vi "UHR-Fleezers Control (host) - 10.6.vi"() -> ()   [LabVIEW 2011] (continued)
      w2669 = T17 0 items=["Grayscale (U8)", "Grayscale (I16)", "Grayscale (SGL)", "Complex (CSG)", "RGB (U32)", "HSL (U32)", "RGB (U64)"] ("Image Type")
      n1729 = for "Create Greyscale map" {
        N: 256 -> [_]
        tunnel: [w2675] -> w2658 mode=indexing
        workers-P: _ -> [_]
        i -> [w2678]
        n1730 = To Unsigned Byte Integer(number=w2678) -> (unsigned 8bit integer=w2674:u8)
        n1731 = Join Numbers(hi=w2674, lo=w2674) -> ((hi.lo)=w2677:u16)
        n1732 = Join Numbers(hi=w2674, lo=w2674) -> ((hi.lo)=w2676:u16)
        n1733 = Join Numbers(hi=w2677, lo=w2676) -> ((hi.lo)=w2675:u32)
      }
      n1734 = call "IMAQ Create"("Image Name"="Scaled video", "Image Type"=w2661) -> ("New Image"=w2660:T2)  [unwired: 2 in, 2 out]
      n1735 = call "IMAQ Create"("Image Name"="Main video", "Image Type"=w2669) -> ("New Image"=w2670:T2)  [unwired: 2 in, 2 out]
      n1736 = node-c288(0 ("Processor")) -> (w2668:T21)  [unwired: 3 out]
      n1737 = Initialize Array(u32 0 ("Window Number (0...15)"), 480 ("dimension size"), 640 ("dimension size")) -> (w2663:u32[][])
      n1738 = timed-loop {
        tunnel: w2673 -> [w2695]
        tunnel: [w2694] -> w2672
        tunnel: w2670 -> [w2693]
        timing: w2668 -> [_]
        timing-out: [_] -> w2667
        tunnel: w2663 -> [w2682]
        tunnel: w2660 -> [w2680]
        tunnel: w2658 -> [w2679]
        stop <- w2681 stop-if-true
        # "This block performs the \nactual image capture."
        n1739 = node-c288() -> ()  [unwired: 2 out]
        n1740 = local read "Stop All"() -> (w2681:bool)
        n1741 = Reciprocal(x="Video Capture Rate (Hz)") -> (1/x=w2685:dbl)
        n1742 = Multiply(x=w2685, y=1000.0) -> (x*y=w2683:dbl)
        n1743 = call "DMR_ImageRequestWaitFor.vi"("queue number IN"=0, "timeout(ms) IN"=500, "driver handle IN"=w2695) -> ("error code OUT"=w2699:i32, "request number OUT"=w2696:i32, "driver handle OUT"=w2697:i32)
        n1744 = feedback #1(T32 refnum ("Avi Refnum")) -> (w2687:T32)
        n1745 = case shown="True" "New Video File" {
          tunnel: [T32 refnum ("Avi Refnum") w2716] -> w2689
          tunnel: [FALSE TRUE] -> w2690
          tunnel: w2687 -> [_ w2712]
          frame False {
          }
          frame True {
            n1746 = call "Create new save file.vi"("Ext"=".avi" ("string"), "Index In"="Video Index") -> ("Path Out"=w2708:path, "Index Out"=w2709:dbl)  [unwired: 1 in]
            "Path Out" <- w2708
            n1747 = Not Equal?(x=w2712, y=T32 refnum ("Avi Refnum")) -> (x != y?=w2713:bool)
            n1748 = Increment(x=w2709) -> (x+1=w2718:dbl)
            n1749 = case shown="True" w2713 {
              tunnel: w2712 -> [_ w2719]
              frame False {
              }
              frame True {
                n1750 = call "IMAQ AVI Close"("Avi Refnum"=w2719) -> ()  [unwired: 1 in, 10 out]
              }
            }
            n1751 = local write "Video Index"(w2718) -> ()
            n1752 = call "IMAQ AVI Create"("Frames Per Second"=u32 30, "AVI Path"=w2708) -> ("Avi Refnum"=w2716:T32)  [unwired: 5 in, 4 out]
          }
        }
        n1753 = Equal To 0?(x=w2699) -> (x = 0?=w2698:bool)
        n1754 = Select(t=w2689, s=w2690, f=w2687) -> (s? t:f=w2688:T32)
        n1755 = feedback-in #1(w2688) -> ()
        n1756 = case shown="True" w2698 {
          tunnel: w2697 -> [w2720 w2745]
          tunnel: w2696 -> [_ w2744]
          tunnel: [w2720 w2741] -> w2694
          tunnel: w2693 -> [_ w2725]
          tunnel: w2682 -> [_ w2729]
          tunnel: w2688 -> [_ w2727]
          tunnel: w2680 -> [_ w2722]
          tunnel: w2679 -> [_ w2721]
          frame False {
          }
          frame True {
            w2735 = u32 0 ("X-offset IN")
            n1757 = call "DMR_GetImageRequestBufferData.vi"("driver handle IN"=w2745, "request number IN"=w2744) -> ("width OUT"=w2734:i32, "height OUT"=w2733:i32, "driver handle OUT"=w2740:i32, "request number OUT"=w2739:i32, "bytes per pixel OUT"=w2736:i32)  [unwired: 13 out]
            n1758 = call "DMR_GetImageRequestBufferImageData.vi"("driver handle IN"=w2740, "request number IN"=w2739, "bytes per pixel IN"=w2736, "X-offset IN"=w2735, "Y-offset IN"=w2735, "height IN"=w2733, "width IN"=w2734) -> ("driver handle OUT"=w2738:u32, "request number OUT"=w2737:u32, "image OUT"=w2730:u32[][])  [unwired: 10 out]
            n1759 = call "DMR_ImageRequestUnlock.vi"("request number IN"=w2737, "driver handle IN"=w2738) -> ("driver handle OUT"=w2743:i32)  [unwired: 1 in, 2 out]
            n1760 = case shown="True" "Averaging" {
              tunnel: w2730 -> [w2781 w2786]
              tunnel: [w2781 w2785] -> w2726
              tunnel: w2729 -> [_ w2783]
              frame False {
              }
              frame True {
                (unwired) 1
                w2791 = 1
                n1761 = feedback #2(w2783) -> (w2782:u32[][])
                n1762 = Add(x=w2786, y=w2782) -> (x+y=w2787:u32[][])
                n1763 = Select(t=w2783, s="Reset Averaging", f=w2787) -> (s? t:f=w2789:u32[][])
                n1764 = feedback-in #2(w2789) -> ()
                n1765 = feedback #3(w2791) -> (w2784:i32)
                n1766 = Divide(x=w2787, y=w2784) -> (x/y=w2788:dbl[][])
                n1767 = Increment(x=w2784) -> (x+1=w2792:i32)
                n1768 = To Unsigned Long Integer(number=w2788) -> (unsigned 32bit integer=w2785:u32[][])
                n1769 = Select(t=w2791, s="Reset Averaging", f=w2792) -> (s? t:f=w2790:i32)
                n1770 = feedback-in #3(w2790) -> ()
              }
            }
            n1771 = call "DMR_ImageRequestSingle.vi"("request control IN"=0, "driver handle IN"=w2743) -> ("driver handle OUT"=w2741:i32)  [unwired: 3 out]
            n1772 = disable-structure shown="Disabled" {
              disable-tunnel: w2726 -> [w2758 _]
              disable-tunnel: w2722 -> [w2757 _]
              frame Disabled {
                n1773 = To Double Precision Float(number=w2758) -> (double precision float=w2756:dbl[][])
                n1774 = In Range and Coerce(upper limit="Intensity Upper", x=w2756, lower limit="Intensity Lower") -> (coerced(x)=w2755:dbl[][])  [unwired: 1 out]
                n1775 = Subtract(x="Intensity Upper", y="Intensity Lower") -> (x-y=w2752:dbl)
                n1776 = Subtract(x=w2755, y="Intensity Lower") -> (x-y=w2753:dbl[][])
                n1777 = Divide(x=w2753, y=w2752) -> (x/y=w2754:dbl[][])
                n1778 = Multiply(x=255.0, y=w2754) -> (x*y=w2750:dbl[][])
                n1779 = To Unsigned Byte Integer(number=w2750) -> (unsigned 8bit integer=w2759:u8[][])
                n1780 = call "IMAQ ArrayToImage"("Image Pixels (U8)"=w2759, "Image"=w2757) -> ("Image Out"=w2746:T2)  [unwired: 4 in, 5 out]
                n1781 = First Call?() -> (First Call?: T/F=w2747:bool)
                n1782 = case shown="True" w2747 {
                  tunnel: w2746 -> [w2760 w2771]
                  frame False {
                    n1783 = flat-sequence {
                      tunnel: w2760 -> [w2766]
                      frame #0 {
                        w2763 = FALSE ("Get/Set Status? (Set)")
                        w2762 = 0 ("Window Number (0...15)")
                        n1784 = call "IMAQ WindSize"("Get/Set Status? (Set)"=w2763, "Window Number"=w2762) -> ("Width & Height out"=→"Window Size":cluster{"Width":i32, "Height":i32})  [unwired: 4 in, 2 out]
                        n1785 = call "IMAQ WindMove"("Window Number (0...15)"=w2762, "Get/Set Status? (Set)"=w2763) -> ("Coordinates (screen)"=→"Window Position":cluster{"X Position":i32, "Y Position":i32})  [unwired: 3 in, 1 out]
                        n1786 = call "IMAQ WindDraw"("Resize to Image Size? (Y)"=FALSE, "Window Number (0...15)"=w2762, "Image"=w2766) -> ()  [unwired: 7 in, 2 out]
                      }
                      frame #1 {
                        n1787 = call "IMAQ WindZoom 2"("Center Point"="Center Point", "Zoom to Fit? (False)"=FALSE, "Zoom Factor"="Zoom Factor") -> ()  [unwired: 5 in, 4 out]
                      }
                    }
                  }
                  frame True {
                    n1788 = flat-sequence {
                      tunnel: w2771 -> [w2774]
                      tunnel: [w2772] -> w2770
                      tunnel: w2770 -> [w2776]
                      frame #0 {
                        w2773 = TRUE ("Resize to Image Size? (Y)")
                        w2772 = 0 ("Window Number (0...15)")
                        n1789 = call "IMAQ WindNonTearing"("Window Number"=w2772, "NonTearing? (True)"=w2773) -> ()  [unwired: 8 in, 2 out]
                        n1790 = call "IMAQ WindDraw"("Resize to Image Size? (Y)"=w2773, "Window Number (0...15)"=w2772, "Image"=w2774) -> ()  [unwired: 7 in, 2 out]
                      }
                      frame #1 {
                        n1791 = call "IMAQ WindSize"("Scrollbars? (N)"=FALSE, "Width & Height"="Initial Window Size", "Window Number"=w2776) -> ()  [unwired: 3 in, 3 out]
                        n1792 = call "IMAQ WindMove"("Window Number (0...15)"=w2776, "Coordinates (screen)"="Initial Window Position") -> ()  [unwired: 3 in, 2 out]
                      }
                    }
                  }
                }
              }
              frame Enabled {
              }
            }
            n1793 = To Unsigned Byte Integer(number=w2726) -> (unsigned 8bit integer=w2724:u8[][])
            n1794 = call "IMAQ ArrayToImage"("Image Pixels (U8)"=w2724, "Image"=w2725) -> ("Image Out"=w2723:T2)  [unwired: 4 in, 5 out]
            "Primary Video Display" <- w2723
            n1795 = case shown="True" "Save Video" {
              tunnel: w2727 -> [_ w2780]
              tunnel: w2723 -> [_ w2779]
              frame False {
              }
              frame True {
                n1796 = call "IMAQ AVI Write Frame"("Image"=w2779, "Avi Refnum"=w2780) -> ()  [unwired: 2 in, 8 out]
              }
            }
            n1797 = case shown="True" "Save Image" {
              tunnel: w2724 -> [_ w2795]
              tunnel: w2721 -> [_ w2794]
              frame False {
              }
              frame True {
                n1798 = call <vilib>:"Flatten Pixmap.vi"("colors"=w2794, "8-bit pixmap"=w2795) -> ("image data"=w2801:T33)  [unwired: 4 in, 5 out]
                n1799 = call "Create new save file.vi"("Insert"="video_frame_" ("string"), "Ext"=".bmp" ("string"), "Index In"="Image Index") -> ("Path Out"=w2797:path, "Index Out"=w2802:dbl)
                n1800 = Increment(x=w2802) -> (x+1=w2796:dbl)
                n1801 = local write "Image Index"(w2796) -> ()
                n1802 = call <vilib>:"Write BMP File.vi"("image data"=w2801, "path to BMP file"=w2797) -> ()  [unwired: 1 in, 9 out]
              }
            }
          }
        }
        n1803 = node-c288(w2683) -> ()  [unwired: 1 out]
      }
      n1804 = node-c288(w2667) -> ()  [unwired: 1 out]
      n1805 = call "DMR_CloseDevice.vi"("driver handle IN"=w2672) -> ()  [unwired: 1 in, 4 out]
    }
    frame #4 {
      n1806 = call "DMR_Close.vi"() -> ()  [unwired: 1 out]
    }
  }
  n1807 = node-c288(i64 1 ("Period"), 1 ("Processor")) -> (w175:T21)  [unwired: 2 out]
  n1808 = timed-loop "Acquire Data" {
    tunnel: w50 -> [w3101]
    tunnel: w49 -> [w3100]
    tunnel: [w3130] -> w270
    tunnel: [w3125] -> w268
    timing: w175 -> [_]
    timing-out: [_] -> w174
    tunnel: w69 -> [w2938]
    stop <- "Stop All" stop-if-true
    w2853 = "Initialize"
    w2923 = "NI_ChannelName" ("name")
    n1809 = node-c288() -> ()  [unwired: 2 out]
    n1810 = First Call?() -> (First Call?: T/F=w2888:bool)
    n1811 = Or(x="Reset", y=w2888) -> (x .or. y?=w2889:bool)
    n1812 = local read "Flushing P1"() -> (w2807:bool)
    n1813 = case "Reset data stream" shown="True" w2889 {
      tunnel: w3101 -> [w4106 w4114]
      tunnel: w3100 -> [w4105 w4113]
      tunnel: [w4106 w4108] -> w3096
      tunnel: [w4105 w4107] -> w3095
      frame False {
      }
      frame True {
        w4111 = TRUE ("AI to FIFO")
        n1814 = local write "Overflow (data lost)"(FALSE ("Overflow (data lost)")) -> ()
        n1815 = call "reset FPGA DMA.vi"("error in"=w4113, "FPGA VI Reference In"=w4114) -> ("error out"=w4109:errorcluster, "FPGA VI Reference Out"=w4110:T19)
        n1816 = xnode "Read/Write Control"("FPGA VI Reference In"=w4110, "error in"=w4109, "AI to FIFO"=w4111, "APD to FIFO"=w4111) -> ("FPGA VI Reference Out"=w4108:T19, "error out"=w4107:errorcluster)
      }
    }
    n1817 = case shown="True" w2807 {
      frame False {
      }
      frame True {
        n1818 = local read "Flush rate (uL/m) P1"() -> (w3147:dbl)
        n1819 = local read "HP1 Flush Time (s)"() -> (w3156:dbl)
        n1820 = local read "DMA Update Period (s)"() -> (w3150:dbl)
        n1821 = Divide(x=w3147, y=60.0) -> (x/y=w3148:dbl)
        n1822 = Divide(x=w3156, y=w3150) -> (x/y=w3145:dbl)
        n1823 = feedback #4(0) -> (w3154:i32)
        n1824 = Increment(x=w3154) -> (x+1=w3144:i32)
        n1825 = Greater?(x=w3144, y=w3145) -> (0:w3153:bool)
        n1826 = Compound Arithmetic op=MULTIPLY(w3150, w3144, w3148) -> (→"P1 Flush Volume (uL)":dbl)
        n1827 = Divide(x=w3144, y=w3145) -> (x/y=→"P1 Flushing Bar":dbl)
        n1828 = case shown="True" w3153 {
          tunnel: w3144 -> [w3157 _]
          tunnel: [w3157 0] -> w3152
          frame False {
          }
          frame True {
            w3158 = FALSE ("Flushing P1")
            n1829 = local write "Inject Pump 1"(w3158) -> ()
            n1830 = local write "Flushing P1"(w3158) -> ()
            n1831 = property on="Clear Volume P1" class="Bool (strict)"("Val(Sgnl)"=TRUE ("Value (Signaling)")) -> ()  [unwired: 2 in, 2 out]
          }
        }
        n1832 = feedback-in #4(w3152) -> ()
      }
    }
    n1833 = Or(x="Start AOD Scan", y="Trap Raster Scan") -> (x .or. y?=w3046:bool)
    n1834 = case "Start AOM raster scan" shown="True" w3046 {
      tunnel: w3096 -> [w3956 w3966]
      tunnel: w3095 -> [w3955 w3965]
      tunnel: [w3956 w3959] -> w3094
      tunnel: [w3955 w3958] -> w3093
      frame False {
      }
      frame True {
        n1835 = case shown="True" "Restart DMA? (AOD)" {
          tunnel: [w4004 w4006] -> w3960
          tunnel: [w4003 w4005] -> w3961
          tunnel: w3966 -> [w4004 w4008]
          tunnel: w3965 -> [w4003 w4007]
          frame False {
          }
          frame True {
            n1836 = local write "Overflow (data lost)"(FALSE ("Overflow (data lost)")) -> ()
            n1837 = call "reset FPGA DMA.vi"("error in"=w4007, "FPGA VI Reference In"=w4008) -> ("error out"=w4005:errorcluster, "FPGA VI Reference Out"=w4006:T19)
          }
        }
        n1838 = local write "Trap Raster Scan"(FALSE ("Trap Raster Scan")) -> ()
        n1839 = case shown="True" "Move MCL Also?" {
          tunnel: w3961 -> [w3969 w3998]
          tunnel: w3960 -> [w3970 w3999]
          tunnel: [w3968 w4002] -> w3959
          tunnel: [w3967 w4001] -> w3958
          frame False {
            w3971 = TRUE ("AI to FIFO")
            n1840 = xnode "Read/Write Control"("FPGA VI Reference In"=w3970, "error in"=w3969, "AI to FIFO"=w3971, "APD to FIFO"=w3971, "Start scan"=w3971) -> ("FPGA VI Reference Out"=w3968:T19, "error out"=w3967:errorcluster)
          }
          frame True {
            w3995 = FALSE ("1D or 2D Scan?")
            w4000 = TRUE ("AI to FIFO")
            # "Count for MCL loop"
            # "N total cycles"
            # "N steps"
            # "V_int"
            n1841 = local read "Scan Range (nm)"() -> (w3977:dbl)
            n1842 = local read "Number of F/B Scans (AOD)"() -> (w3994:u16)
            n1843 = Sign(1:w3977) -> (0:w3976:dbl)
            n1844 = Compound Arithmetic op=MULTIPLY(w3977, "MCL Step Position Ratio", "MCL/AOM Scale Tweak") -> (w3981:dbl)
            n1845 = Negate(x=w3976) -> (-x=w3973:dbl)
            n1846 = Multiply(x=w3973, y="MCL Step Increment (V_int)") -> (x*y=w3975:dbl)
            n1847 = Divide(x=w3981, y="MCL X Cal (nm/V)") -> (x/y=w3987:dbl)
            n1848 = Multiply(x=32767.0 ("y"), y=w3987) -> (x*y=w3993:dbl)
            n1849 = local read "Total Counts (ticks)"() -> (w3978:u32)
            n1850 = local read "Cycles/step (AOD)"() -> (w3989:u64)
            n1851 = local read "Scan steps (AOD)"() -> (w3990:u64)
            n1852 = Divide(x=w3993, y=10.0) -> (x/y=w3986:dbl)
            n1853 = Divide(x=w3986, y="MCL Step Increment (V_int)") -> (x/y=w3984:dbl)
            n1854 = Absolute Value(x=w3984) -> (abs(x)=w3972:dbl)
            n1855 = Compound Arithmetic op=MULTIPLY(w3990, w3989, w3978) -> (w3985:u64)
            n1856 = local write "wait to reset values"(w4000) -> ()
            n1857 = local write "MCL Scanning"(w4000) -> ()
            n1858 = Divide(x=w3985, y=w3972) -> (x/y=w3982:dbl)
            "MCL Count" <- w3982
            n1859 = xnode "Read/Write Control"("FPGA VI Reference In"=w3999, "error in"=w3998, "Scan steps (MCL)"=w3972, "Number of scans (MCL)"=w3994, "Cycles per step (MCL)"=u64 1, "Scan freq.  increment (MCL)"=w3975, "1D or 2D Scan?"=w3995, "MCL Scan Axis"=w3995, "Cont. Scan (MCL)"=w3995, "MCL count"=w3982) -> ("FPGA VI Reference Out"=w3997:T19, "error out"=w3996:errorcluster)
            n1860 = xnode "Read/Write Control"("FPGA VI Reference In"=w3997, "error in"=w3996, "AI to FIFO"=w4000, "APD to FIFO"=w4000, "Start scan"=w4000, "Start scan (MCL)"=w4000) -> ("FPGA VI Reference Out"=w4002:T19, "error out"=w4001:errorcluster)
          }
        }
        "Raster Scanning..." <- TRUE ("Scanning...")
      }
    }
    n1861 = local read "Flushing P3"() -> (w2808:bool)
    n1862 = case "Keep track of when Harvard Pump 3 is done flushing" shown="True" w2808 {
      frame False {
      }
      frame True {
        n1863 = local read "Flush rate (uL/m) P3"() -> (w3164:dbl)
        n1864 = local read "DMA Update Period (s)"() -> (w3166:dbl)
        n1865 = local read "HP3 Flush Time (s)"() -> (w3173:dbl)
        n1866 = Divide(x=w3164, y=60.0) -> (x/y=w3162:dbl)
        n1867 = feedback #5(0) -> (w3171:i32)
        n1868 = Increment(x=w3171) -> (x+1=w3165:i32)
        n1869 = Divide(x=w3173, y=w3166) -> (x/y=w3167:dbl)
        n1870 = Greater?(x=w3165, y=w3167) -> (0:w3170:bool)
        n1871 = Compound Arithmetic op=MULTIPLY(w3166, w3165, w3162) -> (→"P3 Flush Volume (uL)":dbl)
        n1872 = case shown="True" w3170 {
          tunnel: w3165 -> [w3174 _]
          tunnel: [w3174 0] -> w3169
          frame False {
          }
          frame True {
            w3175 = FALSE ("Flushing P3")
            n1873 = local write "Inject Pump 3"(w3175) -> ()
            n1874 = local write "Flushing P3"(w3175) -> ()
            n1875 = property on="Clear Volume P3" class="Bool (strict)"("Val(Sgnl)"=TRUE ("Value (Signaling)")) -> ()  [unwired: 2 in, 2 out]
          }
        }
        n1876 = feedback-in #5(w3169) -> ()
        n1877 = Divide(x=w3165, y=w3167) -> (x/y=→"P3 Flushing Bar":dbl)
      }
    }
    n1878 = And(x="Save scans", y=w3046) -> (x .and. y?=w3092:bool)
    n1879 = Compound Arithmetic op=OR("Start MCL Scan", "Confocal Image", "Confocal Linescan") -> (w3044:bool)
    n1880 = And(x="Save Data (MCL)", y=w3044) -> (x .and. y?=w3091:bool)
    n1881 = case "Start MCL raster scan" shown="True" w3044 {
      tunnel: w3094 -> [w3573 w3589]
      tunnel: w3093 -> [w3572 w3588]
      tunnel: [w3573 w3584] -> w2936
      tunnel: [w3572 w3583] -> w2935
      tunnel: [FALSE w3582] -> w3077
      tunnel: "Start MCL Scan" -> [_ w3577]
      tunnel: "Confocal Image" -> [_ w3576]
      tunnel: "Confocal Linescan" -> [_ _]
      frame False {
      }
      frame True {
        w3582 = TRUE
        n1882 = case shown="True" "Restart DMA? (MCL)" {
          tunnel: [w3634 w3636] -> w3587
          tunnel: [w3633 w3635] -> w3586
          tunnel: w3589 -> [w3634 w3639]
          tunnel: w3588 -> [w3633 w3638]
          frame False {
          }
          frame True {
            n1883 = call "reset FPGA DMA.vi"("error in"=w3638, "FPGA VI Reference In"=w3639) -> ("error out"=w3635:errorcluster, "FPGA VI Reference Out"=w3636:T19)
            n1884 = local write "Overflow (data lost)"(FALSE ("Overflow (data lost)")) -> ()
          }
        }
        n1885 = case shown="False" w3577 {
          selector: w3577 -> [_ w3593]
          tunnel: w3576 -> [w3592 _]
          tunnel: [w3592 w3593] -> w3575
          frame False {
            n1886 = property on="2D or 1D Scan" class="Bool (strict)"("Val(Sgnl)"=w3592) -> ()  [unwired: 2 in, 2 out]
            n1887 = property on="Confocal Image" class="Bool (strict)"("Value"=FALSE ("Start Confocal Map")) -> ()  [unwired: 2 in, 2 out]
          }
          frame True {
          }
        }
        n1888 = local write "MCL Scanning"(w3582) -> ()
        n1889 = local read "AO1"() -> (w3579:dbl)
        n1890 = local read "AO2"() -> (w3578:dbl)
        n1891 = case shown="True" "Center Scan" {
          tunnel: w3587 -> [w3600 w3632]
          tunnel: w3586 -> [w3599 w3631]
          tunnel: [w3598 w3630] -> w3584
          tunnel: [w3597 w3629] -> w3583
          tunnel: [w3595 w3616] -> w3581
          tunnel: [w3594 w3615] -> w3580
          tunnel: w3579 -> [w3595 w3621]
          tunnel: w3578 -> [w3594 w3624]
          tunnel: w3575 -> [_ _]
          frame False {
            w3596 = TRUE ("AI to FIFO")
            n1892 = xnode "Read/Write Control"("FPGA VI Reference In"=w3600, "error in"=w3599, "AI to FIFO"=w3596, "APD to FIFO"=w3596, "Start scan (MCL)"=w3596) -> ("FPGA VI Reference Out"=w3598:T19, "error out"=w3597:errorcluster)
          }
          frame True {
            w3628 = TRUE ("AI to FIFO")
            n1893 = local read "Scan steps (MCL)"() -> (w3607:u64)
            n1894 = local read "Scan lines (y)"() -> (w3603:u64)
            n1895 = local read "Fast Scan Dir"() -> (w3614:bool)
            n1896 = local read "Actual MCL Inc (V)"() -> (w3604:dbl)
            n1897 = Decrement(x=w3603) -> (x-1=w3602:u64)
            n1898 = Decrement(x=w3607) -> (x-1=w3606:u64)
            n1899 = Multiply(x=w3604, y=w3602) -> (x*y=w3601:dbl)
            n1900 = Divide(x=w3601, y=2.0) -> (x/y=w3611:dbl)
            n1901 = Multiply(x=w3604, y=w3606) -> (x*y=w3605:dbl)
            n1902 = Divide(x=w3605, y=2.0) -> (x/y=w3610:dbl)
            n1903 = Select(t=w3610, s=w3614, f=w3611) -> (s? t:f=w3609:dbl)
            n1904 = Select(t=w3611, s=w3614, f=w3610) -> (s? t:f=w3613:dbl)
            n1905 = Subtract(x=w3621, y=w3613) -> (x-y=w3612:dbl)
            n1906 = Subtract(x=w3624, y=w3609) -> (x-y=w3608:dbl)
            n1907 = local read "2D or 1D Scan"() -> (w3626:bool)
            n1908 = Not(x=w3614) -> (.not. x?=w3620:bool)
            n1909 = Not(x=w3626) -> (.not. x?=w3622:bool)
            n1910 = And(x=w3614, y=w3622) -> (x .and. y?=w3623:bool)
            n1911 = And(x=w3622, y=w3620) -> (x .and. y?=w3625:bool)
            n1912 = Select(t=w3624, s=w3625, f=w3608) -> (s? t:f=w3615:dbl)
            n1913 = Select(t=w3621, s=w3623, f=w3612) -> (s? t:f=w3616:dbl)
            n1914 = call "Volt to I16.vi"("Voltage In"=w3616) -> ("I16 Voltage Out"=w3619:i16)
            n1915 = call "Volt to I16.vi"("Voltage In"=w3615) -> ("I16 Voltage Out"=w3618:i16)
            n1916 = xnode "Read/Write Control"("FPGA VI Reference In"=w3632, "error in"=w3631, "AI to FIFO"=w3628, "APD to FIFO"=w3628, "Start scan (MCL)"=w3628, "AO1"=w3619, "AO2"=w3618) -> ("FPGA VI Reference Out"=w3630:T19, "error out"=w3629:errorcluster)
          }
        }
        "Initial Y" <- w3581
        "Initial X" <- w3580
        n1917 = local write "Tab Control 6"(T3."Imaging" ("Tab Control 6")) -> ()
        "wait to reset values" <- w3582
      }
    }
    n1918 = local read "Trap Pos Elements/DMA read"() -> (w2932:u32)
    n1919 = local read "Trap AI Elements/DMA read"() -> (w3007:u32)
    n1920 = local read "APD Elements/DMA read"() -> (w2973:u32)
    n1921 = xnode "Get APD Data"("FPGA VI Reference In"=w2936, "error in"=w2935, "Number of Elements"=w2973, "Timeout (ms)"=-1) -> ("Data"=w2972:u32[], "Elements Remaining"=→"APD FIFO Elements Remaining":u32)  [unwired: 2 out]
    n1922 = xnode "Invoke Method"("FPGA VI Reference In"=w2936, "error in"=w2935, "Number of Elements"=w2932, "Timeout (ms)"=-1) -> ("Data"=w2895:u16[], "Elements Remaining"=→"Trap Pos FIFO El Remaining":u32)  [unwired: 2 out]
    n1923 = xnode "Get Trap Data"("FPGA VI Reference In"=w2936, "error in"=w2935, "Number of Elements"=w3007, "Timeout (ms)"=-1 ("Timeout")) -> ("FPGA VI Reference Out"=w2829:T19, "error out"=w2828:errorcluster, "Data"=w2896:i16[], "Elements Remaining"=w3138:u32)
    "FIFO El. Rem." <- w3138
    n1924 = local read "Trap AI FIFO Depth"() -> (w3140:u32)
    n1925 = Subtract(x=w3140, y=w3007) -> (x-y=w3139:u32)
    n1926 = Decimate 1D Array(w2895) -> (w2892:u16[], w2894:u16[], w2893:u16[])
    n1927 = Divide(x=w3138, y=w3139) -> (x/y=w3137:dbl)
    "Buffer Status" <- w3137
    n1928 = To Unsigned Long Integer(number=w2892) -> (unsigned 32bit integer=w2891:u32[])
    n1929 = Join Numbers(hi=w2894, lo=w2893) -> ((hi.lo)=w2890:u32[])
    n1930 = Equal?(x=w3137, y=1.0) -> (x = y?=w3135:bool)
    n1931 = Join Numbers(hi=w2891, lo=w2890) -> ((hi.lo)=w2884:u64[])
    n1932 = call "IR AOM word to freq - vec.vi"("Frequency Word In (double vec)"=w2884) -> ("Frequency Out"=w2931:dbl[])
    n1933 = case "Alert buffer overflow" shown="True" w3135 {
      frame False {
      }
      frame True {
        n1934 = call <vilib>:"Beep.vi"() -> ()  [unwired: 3 in, 9 out]
        "Overflow (data lost)" <- TRUE ("Overflow (data lost)")
      }
    }
    n1935 = Decimate 1D Array(w2931) -> (w2930:dbl[], w2929:dbl[])
    n1936 = Build Array(w2930, w2929) -> (w2928:dbl[][])
    n1937 = local read "Trap Sets"() -> (w3006:u32)
    n1938 = case "Deinterlace trap data, average down PSD" shown="2" w3006 {
      tunnel: w2896 -> [w3669 w3734]
      tunnel: [w3666 w3731] -> w2999
      tunnel: [w3669 w3733] -> w2887
      tunnel: "Detector Type" -> [w3668 w3729]
      tunnel: [w3667 w3732] -> w2998
      tunnel: [w3665 w3730] -> w3112
      frame 1, Default {
        n1939 = Divide(x=w3669, y=3276.7) -> (x/y=w3670:dbl[])
        n1940 = Decimate 1D Array(w3670) -> (w3679:dbl[], w3678:dbl[], w3677:dbl[], w3676:dbl[], w3675:dbl[], w3674:dbl[], w3673:dbl[], w3672:dbl[])
        n1941 = case shown="\"IR-QPD + PSD + FB-QPD position\"" w3668 {
          tunnel: w3679 -> [w3703 w3728]
          tunnel: w3678 -> [w3702 w3727]
          tunnel: w3677 -> [w3687 w3705]
          tunnel: w3676 -> [w3688 w3715]
          tunnel: w3675 -> [w3701 w3726]
          tunnel: w3674 -> [w3700 w3725]
          tunnel: w3673 -> [w3684 w3706]
          tunnel: w3672 -> [w3683 w3704]
          tunnel: [w3682 w3712] -> w3667
          tunnel: [w3681 w3711] -> w3666
          tunnel: [w3680 w3710] -> w3665
          frame "IR-QPD + PSD + FB-QPD", Default {
            w3680 = 0  # Channel pattern
            n1942 = Divide(x=w3703, y=w3688) -> (x/y=w3690:dbl[])
            n1943 = Divide(x=w3702, y=w3688) -> (x/y=w3689:dbl[])
            n1944 = Divide(x=w3701, y=w3684) -> (x/y=w3686:dbl[])
            n1945 = Divide(x=w3700, y=w3683) -> (x/y=w3685:dbl[])
            n1946 = Build Array(w3690, w3689, w3688, w3687, w3686, w3685, w3684, w3683) -> (w3681:dbl[][])
            n1947 = Bundle("T1 Y", "T1 X", "T1 Sum", "FB Sum", "PSD Y", "PSD X", "PSD Y Sum", "PSD X Sum") -> (w3699:T40)  [unwired: 1 out]
            n1948 = Cluster To Array(cluster=w3699) -> (array=w3682:string[])
          }
          frame "IR-QPD + PSD + FB-QPD position" {
            w3710 = 3  # Channel pattern
            n1949 = Negate(x=w3706) -> (-x=w3707:dbl[])
            n1950 = Divide(x=w3728, y=w3715) -> (x/y=w3717:dbl[])
            n1951 = Divide(x=w3727, y=w3715) -> (x/y=w3716:dbl[])
            n1952 = Divide(x=w3726, y=w3706) -> (x/y=w3714:dbl[])
            n1953 = Divide(x=w3725, y=w3707) -> (x/y=w3713:dbl[])
            n1954 = Build Array(w3717, w3716, w3715, w3704, w3705, w3714, w3713, w3706) -> (w3711:dbl[][])
            n1955 = Bundle("T1 Y", "T1 X", "T1 Sum", "FB X", "FB Sum", "PSD Y", "PSD X", "PSD Y Sum") -> (w3724:T40)  [unwired: 1 out]
            n1956 = Cluster To Array(cluster=w3724) -> (array=w3712:string[])
          }
        }
      }
      frame 2 {
        n1957 = case shown="\"IR-QPD + PSD + FB-QPD X position\"" w3729 {
          tunnel: w3734 -> [w3796 w3863 w3934]
          tunnel: [w3735 w3854 w3865] -> w3733
          tunnel: [w3762 w3845 w3912] -> w3732
          tunnel: [w3761 w3808 w3879] -> w3731
          tunnel: [w3755 w3843 w3910] -> w3730
          frame "IR-QPD + PSD + FB-QPD", Default {
            w3755 = 1  # Channel pattern
            # "time average x2 the 4th signal and the 4 psd signals (detection laser)"
            # "deinterlace 3 signals from qpd"
            n1958 = Decimate 1D Array(w3796) -> (w3795:i16[], w3794:i16[], w3760:i16[], w3793:i16[], w3783:i16[], w3781:i16[], w3780:i16[], w3778:i16[])
            n1959 = Decimate 1D Array(w3760) -> (w3759:i16[], w3758:i16[])
            n1960 = Decimate 1D Array(w3795) -> (w3792:i16[], w3764:i16[])
            n1961 = Decimate 1D Array(w3794) -> (w3791:i16[], w3789:i16[])
            n1962 = Decimate 1D Array(w3793) -> (w3790:i16[], w3788:i16[])
            n1963 = call "downsample 1D array - double.vi"("Ave N"=2.0, "Array In"=w3783) -> ("Array Out"=w3782:dbl[])  [unwired: 1 out]
            n1964 = call "downsample 1D array - double.vi"("Ave N"=2.0, "Array In"=w3781) -> ("Array Out"=w3763:dbl[])  [unwired: 1 out]
            n1965 = call "downsample 1D array - double.vi"("Ave N"=2.0, "Array In"=w3780) -> ("Array Out"=w3779:dbl[])  [unwired: 1 out]
            n1966 = call "downsample 1D array - double.vi"("Ave N"=2.0, "Array In"=w3778) -> ("Array Out"=w3777:dbl[])  [unwired: 1 out]
            n1967 = Interleave 1D Arrays(w3792, w3791, w3790, w3764, w3789, w3788, w3759, w3758, w3782, w3763, w3779, w3777) -> (w3776:dbl[])
            n1968 = Divide(x=w3776, y=3276.7) -> (x/y=w3775:dbl[])
            n1969 = Decimate 1D Array(w3775) -> (w3774:dbl[], w3773:dbl[], w3772:dbl[], w3771:dbl[], w3770:dbl[], w3769:dbl[], w3757:dbl[], w3756:dbl[], w3768:dbl[], w3767:dbl[], w3766:dbl[], w3765:dbl[])
            n1970 = Divide(x=w3774, y=w3772) -> (x/y=w3742:dbl[])
            n1971 = Divide(x=w3773, y=w3772) -> (x/y=w3741:dbl[])
            n1972 = Divide(x=w3771, y=w3769) -> (x/y=w3740:dbl[])
            n1973 = Divide(x=w3770, y=w3769) -> (x/y=w3739:dbl[])
            n1974 = Divide(x=w3768, y=w3766) -> (x/y=w3738:dbl[])
            n1975 = Divide(x=w3767, y=w3765) -> (x/y=w3737:dbl[])
            n1976 = Build Array(w3742, w3741, w3772, w3740, w3739, w3769, w3757, w3756, w3738, w3737, w3766, w3765) -> (w3761:dbl[][])
            n1977 = Bundle("T1 Y", "T1 X", "T1 Sum", "T2 Y", "T2 X", "T2 Sum", "T1 FB Sum", "T2 FB Sum", "PSD Y", "PSD X", "PSD Y Sum", "PSD X Sum") -> (w3743:T41)  [unwired: 1 out]
            n1978 = To Word Integer(number=w3776) -> (16bit integer=w3735:i16[])
            n1979 = Cluster To Array(cluster=w3743) -> (array=w3762:string[])
          }
          frame "IR-QPD + PSD + FB-QPD X position" {
            w3843 = 2  # Channel pattern
            # "time average x2 the 3 psd signals (detection laser)"
            # "deinterlace 3 signals from qpds"
            n1980 = Decimate 1D Array(w3863) -> (w3862:i16[], w3861:i16[], w3844:i16[], w3860:i16[], w3806:i16[], w3803:i16[], w3800:i16[], w3831:i16[])
            n1981 = Decimate 1D Array(w3844) -> (w3829:i16[], w3827:i16[])
            n1982 = Decimate 1D Array(w3862) -> (w3859:i16[], w3846:i16[])
            n1983 = Decimate 1D Array(w3861) -> (w3858:i16[], w3856:i16[])
            n1984 = Decimate 1D Array(w3860) -> (w3857:i16[], w3855:i16[])
            n1985 = Decimate 1D Array(w3831) -> (w3830:i16[], w3828:i16[])
            n1986 = call "downsample 1D array - I16.vi"("Ave N"=2.0, "Array In"=w3806) -> ("Array Out"=w3804:i16[])  [unwired: 1 in]
            n1987 = call "downsample 1D array - I16.vi"("Ave N"=2.0, "Array In"=w3800) -> ("Array Out"=w3798:i16[])  [unwired: 1 in]
            n1988 = call "downsample 1D array - I16.vi"("Ave N"=2.0, "Array In"=w3803) -> ("Array Out"=w3801:i16[])  [unwired: 1 in]
            n1989 = Interleave 1D Arrays(w3859, w3858, w3857, w3846, w3856, w3855, w3830, w3829, w3828, w3827, w3804, w3801, w3798) -> (w3854:i16[])
            n1990 = Divide(x=w3854, y=3276.7) -> (x/y=w3853:dbl[])
            n1991 = Decimate 1D Array(w3853) -> (w3852:dbl[], w3851:dbl[], w3850:dbl[], w3849:dbl[], w3848:dbl[], w3847:dbl[], w3819:dbl[], w3817:dbl[], w3816:dbl[], w3814:dbl[], w3813:dbl[], w3812:dbl[], w3809:dbl[])
            n1992 = Negate(x=w3809) -> (-x=w3807:dbl[])
            n1993 = Divide(x=w3813, y=w3809) -> (x/y=w3811:dbl[])
            n1994 = Divide(x=w3812, y=w3807) -> (x/y=w3810:dbl[])
            n1995 = Divide(x=w3852, y=w3850) -> (x/y=w3835:dbl[])
            n1996 = Divide(x=w3851, y=w3850) -> (x/y=w3834:dbl[])
            n1997 = Divide(x=w3849, y=w3847) -> (x/y=w3833:dbl[])
            n1998 = Divide(x=w3848, y=w3847) -> (x/y=w3832:dbl[])
            n1999 = Divide(x=w3819, y=w3817) -> (x/y=w3818:dbl[])
            n2000 = Divide(x=w3816, y=w3814) -> (x/y=w3815:dbl[])
            n2001 = Build Array(w3835, w3834, w3850, w3833, w3832, w3847, w3818, w3817, w3815, w3814, w3811, w3810, w3809) -> (w3808:dbl[][])
            n2002 = Bundle("T1 Y", "T1 X", "T1 Sum", "T2 Y", "T2 X", "T2 Sum", "T1 FB X", "T1 FB Sum", "T2 FB X", "T2 FB Sum", "PSD Y", "PSD X", "PSD Y Sum") -> (w3836:T42)  [unwired: 1 out]
            n2003 = Cluster To Array(cluster=w3836) -> (array=w3845:string[])
          }
          frame "IR-QPD + PSD + FB-QPD XY positions" {
            w3910 = 4  # Channel pattern
            # "time average x2 the 3 psd signals (detection laser)"
            # "deinterlace 3 signals from qpds"
            n2004 = Decimate 1D Array(w3934) -> (w3933:i16[], w3932:i16[], w3911:i16[], w3931:i16[], w3877:i16[], w3923:i16[], w3922:i16[], w3899:i16[])
            n2005 = Decimate 1D Array "Feedback Sum"(w3911) -> (w3895:i16[], w3893:i16[])
            n2006 = Decimate 1D Array "QPD Y"(w3933) -> (w3930:i16[], w3913:i16[])
            n2007 = Decimate 1D Array "QPD X"(w3932) -> (w3929:i16[], w3927:i16[])
            n2008 = Decimate 1D Array "Feedback Y"(w3877) -> (w3876:i16[], w3875:i16[])
            n2009 = Decimate 1D Array "QPD Sum"(w3931) -> (w3928:i16[], w3926:i16[])
            n2010 = Decimate 1D Array "Feedback X"(w3899) -> (w3896:i16[], w3894:i16[])
            n2011 = call "downsample 1D array - double.vi"("Ave N"=2.0, "Array In"=w3923) -> ("Array Out"=w3898:dbl[])  [unwired: 1 out]
            n2012 = call "downsample 1D array - double.vi"("Ave N"=2.0, "Array In"=w3922) -> ("Array Out"=w3897:dbl[])  [unwired: 1 out]
            n2013 = Interleave 1D Arrays(w3930, w3929, w3928, w3913, w3927, w3926, w3876, w3896, w3895, w3875, w3894, w3893, w3898, w3897) -> (w3921:dbl[])
            n2014 = Divide(x=w3921, y=3276.7) -> (x/y=w3920:dbl[])
            n2015 = Decimate 1D Array(w3920) -> (w3919:dbl[], w3918:dbl[], w3917:dbl[], w3916:dbl[], w3915:dbl[], w3914:dbl[], w3872:dbl[], w3886:dbl[], w3870:dbl[], w3871:dbl[], w3884:dbl[], w3868:dbl[], w3882:dbl[], w3880:dbl[])
            n2016 = Negate(x=w3880) -> (-x=w3878:dbl[])
            n2017 = Divide(x=w3882, y=w3878) -> (x/y=w3881:dbl[])
            n2018 = Divide(x=w3871, y=w3868) -> (x/y=w3867:dbl[])
            n2019 = Divide(x=w3872, y=w3870) -> (x/y=w3869:dbl[])
            n2020 = Divide(x=w3919, y=w3917) -> (x/y=w3903:dbl[])
            n2021 = Divide(x=w3918, y=w3917) -> (x/y=w3902:dbl[])
            n2022 = Divide(x=w3916, y=w3914) -> (x/y=w3901:dbl[])
            n2023 = Divide(x=w3915, y=w3914) -> (x/y=w3900:dbl[])
            n2024 = Divide(x=w3886, y=w3870) -> (x/y=w3885:dbl[])
            n2025 = Divide(x=w3884, y=w3868) -> (x/y=w3883:dbl[])
            n2026 = Build Array(w3903, w3902, w3917, w3901, w3900, w3914, w3869, w3885, w3870, w3867, w3883, w3868, w3881, w3880) -> (w3879:dbl[][])
            n2027 = Bundle("T1 Y", "T1 X", "T1 Sum", "T2 Y", "T2 X", "T2 Sum", "T1 FB Y", "T1 FB X", "T1 FB Sum", "T2 FB Y", "T2 FB X", "T2 FB Sum", "PSD X", "PSD Y Sum") -> (w3866:T43)  [unwired: 1 out]
            n2028 = To Word Integer(number=w3921) -> (16bit integer=w3865:i16[])
            n2029 = Cluster To Array(cluster=w3866) -> (array=w3912:string[])
          }
        }
      }
    }
    "AI labels" <- w2998
    n2030 = Decimate 1D Array(w2972) -> (w2996:u32[], w2940:u32[])
    n2031 = local read "DMA Update Period (s)"() -> (w3008:dbl)
    n2032 = Build Array(w2996, w2940) -> (w3074:u32[][])
    n2033 = local read "Data Period (s)"() -> (w2846:dbl)
    n2034 = local read "BD 1 Frequency 2 (MHz)"() -> (w2879:dbl)
    n2035 = local read "BD 1 Frequency 1 (MHz)"() -> (w2880:dbl)
    n2036 = Decimate 1D Array(w2887) -> (w2911:i16[], w2910:i16[], w2908:i16[], w2907:i16[])  [unwired: 9 out]
    n2037 = To Double Precision Float(number=w3074) -> (double precision float=w3075:dbl[][])
    n2038 = local read "APD Integration Time (s)"() -> (w2953:dbl)
    n2039 = Multiply(x=w2846, y="Trap Pos. Disp. Downsample") -> (x*y=w2844:dbl)
    n2040 = Divide(x=w2911, y=w2910) -> (x/y=w2912:dbl[])
    n2041 = Divide(x=w2908, y=w2907) -> (x/y=w2909:dbl[])
    n2042 = feedback #6(0.0) -> (w2925:dbl)
    n2043 = Add(x=w3008, y=w2925) -> (x+y=w3114:dbl)
    n2044 = feedback-in #6(w3114) -> ()
    n2045 = local read "AOM X Cal (nm/MHz)"() -> (w2877:dbl)
    n2046 = To Time Stamp(1:w2925) -> (0:w2924:timestamp)
    n2047 = Split 1D Array(array=w2912, index="N El. to Ave.") -> (second subarray=w2915:dbl[])  [unwired: 1 out]
    n2048 = Split 1D Array(array=w2909, index="N El. to Ave.") -> (second subarray=w2914:dbl[])  [unwired: 1 out]
    n2049 = Multiply(x=w2846, y="Trap Disp. Downsample") -> (x*y=w2926:dbl)
    "Display Period (s)" <- w2926
    n2050 = for "Trap AI" {
      tunnel: [w3664] -> w3108 mode=indexing
      tunnel: w2924 -> [w3654]
      tunnel: "Trap Disp. Downsample" -> [w3662]
      tunnel: w2999 -> [w3660] mode=indexing
      tunnel: w2846 -> [w3659]
      tunnel: w2998 -> [w3658] mode=indexing
      tunnel: w2923 -> [w3657]
      tunnel: [w3656] -> w2964 mode=indexing
      tunnel: w2926 -> [w3655]
      workers-P: _ -> [_]
      n2051 = Bundle By Name("Y"=w3660, "dt"=w3659) -> (w3661:waveform(dbl))  [unwired: 1 out]
      n2052 = Set Waveform Attribute(5:w3658, 6:w3657, 7:w3661) -> (3:w3656:waveform(dbl))  [unwired: 1 in, 2 out]
      n2053 = call "downsample 1D array - double.vi"("Ave N"=w3662, "Array In"=w3660) -> ("Array Out"=w3663:dbl[])  [unwired: 1 out]
      n2054 = Bundle By Name(cluster=w3656, "t0"=w3654, "Y"=w3663, "dt"=w3655) -> (w3664:waveform(dbl))
    }
    n2055 = Bundle("BD 1 Frequency 1 (MHz)"=w2880, "BD 1 Frequency 2 (MHz)"=w2879) -> (w2881:T44)  [unwired: 1 out]
    n2056 = call <vilib>:"Mean.vi"("X"=w2914) -> ("mean"=w2902:dbl)  [unwired: 1 out]
    n2057 = call <vilib>:"Mean.vi"("X"=w2915) -> ("mean"=w2903:dbl)  [unwired: 1 out]
    n2058 = Reciprocal(x=w2926) -> (1/x=→"Trap Disp. Freq. (Hz)":dbl)
    n2059 = Cluster To Array(cluster=w2881) -> (array=w2878:dbl[])
    n2060 = local read "Trap X AI1 (DMA)"() -> (w2913:T13)
    n2061 = local read "Data points/scans (MCL)"() -> (w3086:dbl)
    n2062 = To Fixed-Point(number=w2902) -> (fixed-point=w2900:fxp<+/-,16,1>)  [unwired: 1 in]
    n2063 = To Fixed-Point(number=w2903) -> (fixed-point=w2901:fxp<+/-,16,1>)  [unwired: 1 in]
    n2064 = Bundle("Trap 1 Pos.", "Trap 2 Pos.") -> (w2922:cluster{string, string})  [unwired: 1 out]
    n2065 = Bundle By Name(cluster=w2913, "Set 1"=w2901, "Set 2"=w2900) -> (→"Trap X AI1 (DMA)":T13)
    n2066 = Cluster To Array(cluster=w2922) -> (array=w2919:string[])
    n2067 = Bundle("APD 1", "APD 2") -> (w3107:cluster{string, string})  [unwired: 1 out]
    n2068 = Select(t=-1.0, s="Negate Y Axis", f=1.0) -> (s? t:f=w2863:dbl)
    n2069 = for "Trap Position" {
      tunnel: w2928 -> [w3303] mode=indexing
      tunnel: "Trap Pos. Disp. Downsample" -> [w3302]
      tunnel: w2844 -> [w3300]
      tunnel: w2924 -> [w3299]
      tunnel: w2923 -> [w3297]
      tunnel: w2919 -> [w3296] mode=indexing
      tunnel: [w3295] -> w2833 mode=indexing
      tunnel: w2878 -> [w3293] mode=indexing
      tunnel: w2877 -> [w3291]
      tunnel: w2863 -> [w3290]
      n2070 = call "downsample 1D array - double.vi"("Ave N"=w3302, "Array In"=w3303) -> ("Array Out"=w3301:dbl[])  [unwired: 1 out]
      n2071 = Subtract(x=w3301, y=w3293) -> (x-y=w3294:dbl[])
      n2072 = Multiply(x=w3291, y=w3294) -> (x*y=w3292:dbl[])
      n2073 = Multiply(x=w3290, y=w3292) -> (x*y=w3289:dbl[])
      n2074 = Bundle By Name("Y"=w3289, "dt"=w3300, "t0"=w3299) -> (w3298:waveform(dbl))  [unwired: 1 out]
      n2075 = Set Waveform Attribute(5:w3296, 6:w3297, 7:w3298) -> (3:w3295:waveform(dbl))  [unwired: 1 in, 2 out]
    }
    n2076 = Cluster To Array(cluster=w3107) -> (array=w3104:string[])
    n2077 = for "APD" {
      tunnel: w3075 -> [w3643] mode=indexing
      tunnel: w2953 -> [w3651]
      tunnel: [w3647] -> w2960 mode=indexing
      tunnel: "APD Disp. Scale" -> [w3648]
      tunnel: w2923 -> [w3646]
      tunnel: w3104 -> [w3645] mode=indexing
      tunnel: "APD Disp. Downsample" -> [w3641]
      tunnel: [w3644] -> w3103
      workers-P: _ -> [_]
      tunnel: w2924 -> [w3640]
      n2078 = call "integrate 1D array interval - double.vi"("Ave N"=w3641, "Array In"=w3643) -> ("Array Out"=w3642:dbl[])  [unwired: 1 out]
      n2079 = Multiply(x=w3651, y=w3641) -> (x*y=w3644:dbl)
      n2080 = Divide(x=w3642, y=w3648) -> (x/y=w3649:dbl[])
      n2081 = Bundle By Name("t0"=w3640, "Y"=w3649, "dt"=w3644) -> (w3650:waveform(dbl))  [unwired: 1 out]
      n2082 = Set Waveform Attribute(5:w3645, 6:w3646, 7:w3650) -> (3:w3647:waveform(dbl))  [unwired: 1 in, 2 out]
    }
    "APD Display Period (s)" <- w3103
    n2083 = Reciprocal(x=w3103) -> (1/x=→"APD Display Freq. (Hz)":dbl)
    n2084 = local read "Display Period (s)"() -> (w2984:dbl)
    n2085 = Increment(x=w3086) -> (x+1=w3087:dbl)
    n2086 = To Double Precision Float(number=w2996) -> (double precision float=w2995:dbl[])
    n2087 = Index Array(array=w2833, index=0) -> (element=w2837:waveform(dbl))
    n2088 = Index Array(array=w2833, index=1) -> (element=w2832:waveform(dbl))
    n2089 = feedback #7(w3087) -> (w3090:dbl)
    n2090 = Select(t=0, s=w3077, f=w3090) -> (s? t:f=w3083:dbl)
    n2091 = Array Size(array=w2995) -> (size(s)=w3089:i32)
    n2092 = Add(x=w3089, y=w3083) -> (x+y=w3084:dbl)
    n2093 = Unbundle By Name(w2837) -> ("Y"=w2838:dbl[])
    n2094 = feedback #8(w2996) -> (w3073:u32[])
    n2095 = Build Array (concatenate)(w3073, w2996) -> (w3070:u32[])
    n2096 = feedback #9(w2940) -> (w2959:u32[])
    n2097 = Divide(x="Bead Sep. Int. Time (s)", y=w2984) -> (x/y=w2873:dbl)
    n2098 = Build Array (concatenate)(w2959, w2940) -> (w2958:u32[])
    n2099 = Add(x=w2838, y="FB Trap Pos Offset") -> (x+y=w2836:dbl[])
    "T1 x pos data" <- w2836
    n2100 = Greater?(x=w3084, y=w3086) -> (0:w3085:bool)
    n2101 = feedback #10(w2836) -> (w2875:dbl[])
    n2102 = Build Array (concatenate)(w2836, w2875) -> (w2874:dbl[])
    n2103 = Bundle By Name(cluster=w2837, "Y"=w2836) -> (w2835:waveform(dbl))
    n2104 = Select(t=w3083, s=w3085, f=w3084) -> (s? t:f=w3082:dbl)
    n2105 = feedback-in #7(w3082) -> ()
    n2106 = Array Size(array=w3070) -> (size(s)=w3067:i32)
    n2107 = Array Size(array=w2996) -> (size(s)=w3069:i32)
    n2108 = local read "MCL Scanning"() -> (w3080:bool)
    n2109 = local read "APD Integration Time (s)"() -> (w2967:dbl)
    n2110 = Bundle(w2835, w2832) -> (w2831:cluster{waveform(dbl), waveform(dbl)})  [unwired: 1 out]
    n2111 = Build Array (concatenate)(w2960, w3108) -> (w2962:waveform(dbl)[])
    "All Signals" <- w2962
    n2112 = Split 1D Array(array=w2874, index=w2873) -> (first subarray=w2867:dbl[])  [unwired: 1 out]
    n2113 = feedback-in #10(w2867) -> ()
    n2114 = Multiply(x=w3069, y="APD Ave N") -> (x*y=w3068:dbl)
    n2115 = Greater?(x=w3067, y=w3068) -> (0:w3071:bool)
    n2116 = Not(x=w3085) -> (.not. x?=w3079:bool)
    n2117 = Cluster To Array(cluster=w2831) -> (array=→"Trap Positions":waveform(dbl)[])
    n2118 = To Double Precision Float(number=w2940) -> (double precision float=w2939:dbl[])
    n2119 = call <vilib>:"Mean.vi"("X"=w2867) -> ("mean"=w2866:dbl)  [unwired: 1 out]
    "Mean T1 Position (nm)" <- w2866
    n2120 = Subtract(x=w2867, y=w2866) -> (x-y=w2872:dbl[])
    n2121 = Square(x=w2872) -> (x^2=w2871:dbl[])
    n2122 = And(x=w3079, y=w3080) -> (x .and. y?=w3081:bool)
    n2123 = call <vilib>:"Mean.vi"("X"=w2871) -> ("mean"=w2870:dbl)  [unwired: 1 out]
    n2124 = case shown="True" w3071 {
      tunnel: w3070 -> [w3423 w3430]
      tunnel: [w3423 w3428] -> w3013
      tunnel: w3068 -> [_ w3425]
      tunnel: w3067 -> [_ w3429]
      tunnel: w2958 -> [w3422 w3427]
      tunnel: [w3422 w3424] -> w2955
      frame False {
      }
      frame True {
        n2125 = Subtract(x=w3429, y=w3425) -> (x-y=w3426:dbl)
        n2126 = Array Subset(array=w3430, index=w3426, length=w3425) -> (w3428:u32[])
        n2127 = Array Subset(array=w3427, index=w3426, length=w3425) -> (w3424:u32[])
      }
    }
    n2128 = feedback-in #8(w3013) -> ()
    n2129 = feedback-in #9(w2955) -> ()
    n2130 = Square Root(x=w2870) -> (sqrt(x)=w2869:dbl)
    n2131 = Or(x=w3081, y=w3077) -> (x .or. y?=w3078:bool)
    n2132 = Equal?(x="Tab Control 6", y=T34."High Res Display") -> (x = y?=w3002:bool)
    n2133 = Multiply(x="APD Disp. Scale", y=w2960) -> (x*y=w2969:waveform(dbl)[])
    n2134 = Multiply(x=10.0, y=w2869) -> (x*y=→"Trap 1 Position RMS (A)":dbl)
    n2135 = Multiply(x="APD Disp. Downsample", y=w2967) -> (x*y=w2965:dbl)
    n2136 = Divide(x=w2969, y=w2965) -> (x/y=w2937:waveform(dbl)[])
    n2137 = case "For displaying the high resolution display (no downsampling)" shown="True" w3002 {
      tunnel: w2964 -> [_ w3323]
      frame False {
      }
      frame True {
        n2138 = Index Array(array=w3323, index="High Res. Display") -> (element=w3324:waveform(dbl))
        n2139 = call <vilib>:"Std Deviation and Variance.vi"("X"=w3324) -> ("mean"=w3331:dbl, "standard deviation"=w3336:dbl)  [unwired: 1 in, 1 out]
        "Mean Intensity" <- w3331
        "Sigma" <- w3336
        n2140 = Subtract(x=w3324, y=w3331) -> (x-y=w3330:waveform(dbl))
        n2141 = Select(t=w3330, s="Subtract mean", f=w3324) -> (s? t:f=→"1 Channel":waveform(dbl))
        n2142 = Divide(x=w3336, y=w3331) -> (x/y=→"Sigma/Mean":dbl)
        n2143 = feedback #11(1) -> (w3325:i32)
        n2144 = Greater Or Equal?(x=w3325, y="Slow mean N ave.") -> (x >= y?=w3338:bool)
        n2145 = Increment(x=w3325) -> (x+1=w3340:i32)
        n2146 = Select(t=1, s=w3338, f=w3340) -> (s? t:f=w3327:i32)
        n2147 = feedback-in #11(w3327) -> ()
        n2148 = feedback #12() -> (w3328:waveform(dbl))  [unwired: 1 out]
        n2149 = case shown="Default" w3325 {
          tunnel: [w3343 w3346] -> w3329
          tunnel: w3328 -> [w3345 _]
          tunnel: w3324 -> [w3344 w3346]
          frame Default {
            n2150 = call-poly <vilib>:"Append Waveforms.vi"("waveform B"=w3344, "waveform A"=w3345) -> ("waveform out"=w3343:waveform(dbl))  [unwired: 1 in, 8 out]
          }
          frame 1 {
          }
        }
        n2151 = feedback-in #12(w3329) -> ()
        n2152 = case shown="True" w3338 {
          tunnel: w3329 -> [_ w3342]
          frame False {
          }
          frame True {
            n2153 = call <vilib>:"Mean.vi"("X"=w3342) -> ("mean"=→"Slow mean":dbl)  [unwired: 1 out]
          }
        }
      }
    }
    n2154 = Index Array(array=w2937, index=0) -> (element=w2947:waveform(dbl))
    n2155 = Index Array(array=w2937, index=1) -> (element=w2945:waveform(dbl))
    n2156 = case "For computing FFTs for display" shown="True" "Compute FFT" {
      tunnel: w2964 -> [_ w4037]
      frame False {
      }
      frame True {
        n2157 = Build Array("FFT 1 Choice 1", "FFT 1 Choice 2", "FFT 2 Choice 1", "FFT 2 Choice 2") -> (w4030:u16[])
        n2158 = Array Size(array=w4037) -> (size(s)=w4036:i32)
        n2159 = feedback-in #13(w4030) -> ()
        n2160 = feedback #13(u16[] [100, 100, 100, 100]) -> (w4031:u16[])
        n2161 = feedback-in #14("# Spectra to Ave.") -> ()
        n2162 = feedback #14("# Spectra to Ave.") -> (w4028:dbl)
        n2163 = Not Equal?(x="# Spectra to Ave.", y=w4028) -> (x != y?=w4027:bool)
        n2164 = Not Equal?(x=w4030, y=w4031) -> (x != y?=w4029:bool)
        n2165 = feedback #15(1.0) -> (w4014:dbl)
        n2166 = Compound Arithmetic op=OR("Reset FFT", w4029, w4027) -> (w4012:bool)
        n2167 = Select(t=1.0, s=w4012, f=w4014) -> (s? t:f=w4016:dbl)
        n2168 = Greater?(x=w4016, y="# Spectra to Ave.") -> (0:w4035:bool)
        n2169 = Increment(x=w4016) -> (x+1=w4015:dbl)
        n2170 = feedback-in #15(w4015) -> ()
        n2171 = local read "DMA Update Period (s)"() -> (w4010:dbl)
        n2172 = Multiply(x="# Spectra to Ave.", y=w4010) -> (x*y=→"Ave. Time (s)":dbl)
        n2173 = Build Array(cluster{"f0":dbl, "df":dbl, "magnitude":dbl[]} {"f0"=0.0, "df"=0.0, "magnitude"=[]} ("PSD")) -> (w4019:cluster{"f0":dbl, "df":dbl, "magnitude":dbl[]}[])
        n2174 = Build Array(w4019, w4019, w4019, w4019) -> (w4021:T45)
        n2175 = feedback #16(w4021) -> (w4026:T45)
        n2176 = for {
          N: 4 -> [_]
          tunnel: w4030 -> [w4059] mode=indexing
          tunnel: w4037 -> [w4060]
          tunnel: w4036 -> [w4062]
          tunnel: w4012 -> [w4055]
          tunnel: w4035 -> [w4054]
          tunnel: "# Spectra to Ave." -> [w4053]
          tunnel: [w4052] -> w4025 mode=indexing
          tunnel: w4026 -> [w4057] mode=indexing
          tunnel: [w4056] -> w4013 mode=indexing
          tunnel: w4016 -> [w4051]
          n2177 = Less?(x=w4059, y=w4062) -> (x < y?=w4061:bool)
          n2178 = Index Array(array=w4060, index=w4059) -> (element=w4058:waveform(dbl))
          n2179 = case shown="True" w4061 {
            tunnel: w4058 -> [_ w4079]
            tunnel: w4057 -> [w4064 w4077]
            tunnel: [w4064 w4065] -> w4056
            tunnel: w4055 -> [_ w4076]
            tunnel: w4054 -> [_ w4069]
            tunnel: w4053 -> [_ w4068]
            tunnel: [cluster{"f0":dbl, "df":dbl, "magnitude":dbl[]} {"f0"=0.0, "df"=0.0, "magnitude"=[]} ("PSD") w4070] -> w4052
            tunnel: w4051 -> [_ w4067]
            frame False {
            }
            frame True {
              n2180 = call <vilib>:"Std Deviation and Variance.vi"("X"=w4079) -> ("mean"=w4080:dbl)  [unwired: 1 in, 2 out]
              n2181 = Subtract(x=w4079, y=w4080) -> (x-y=w4078:waveform(dbl))
              n2182 = xnode "Spectral Measurements"("Signals"=w4078) -> ("PSD"=w4072:cluster{"f0":dbl, "df":dbl, "magnitude":dbl[]})  [unwired: 1 in, 1 out]
              n2183 = case shown="False" w4076 {
                tunnel: w4077 -> [w4089 _]
                tunnel: [w4085 w4094] -> w4065
                tunnel: w4072 -> [w4088 w4095]
                tunnel: w4069 -> [w4087 _]
                frame False {
                  n2184 = Build Array (concatenate)(w4089, w4088) -> (w4086:cluster{"f0":dbl, "df":dbl, "magnitude":dbl[]}[])
                  n2185 = case shown="True" w4087 {
                    tunnel: w4086 -> [w4090 w4093]
                    tunnel: [w4090 w4091] -> w4085
                    frame False {
                    }
                    frame True {
                      n2186 = Delete From Array(array=w4093, index=0) -> (array with subset deleted=w4091:cluster{"f0":dbl, "df":dbl, "magnitude":dbl[]}[])  [unwired: 1 in, 1 out]
                    }
                  }
                }
                frame True {
                  n2187 = Build Array(w4095) -> (w4094:cluster{"f0":dbl, "df":dbl, "magnitude":dbl[]}[])
                }
              }
              n2188 = for {
                tunnel: w4065 -> [w4084] mode=indexing
                tunnel: [w4083] -> w4075 mode=indexing
                workers-P: _ -> [_]
                n2189 = Unbundle By Name(w4084) -> ("magnitude"=w4083:dbl[])
              }
              n2190 = Transpose 2D Array(2D array=w4075) -> (transposed array=w4074:dbl[][])
              n2191 = for {
                tunnel: w4074 -> [w4082] mode=indexing
                tunnel: [w4081] -> w4073 mode=indexing
                workers-P: _ -> [_]
                n2192 = Add Array Elements(numeric array=w4082) -> (sum=w4081:dbl)
              }
              n2193 = Select(t=w4068, s=w4069, f=w4067) -> (s? t:f=w4066:dbl)
              n2194 = Divide(x=w4073, y=w4066) -> (x/y=w4071:dbl[])
              n2195 = Bundle By Name(cluster=w4072, "magnitude"=w4071) -> (w4070:cluster{"f0":dbl, "df":dbl, "magnitude":dbl[]})
            }
          }
        }
        n2196 = case shown="True" w4012 {
          tunnel: w4013 -> [w4044 w4050]
          tunnel: [w4044 w4045] -> w4011
          frame False {
          }
          frame True {
            n2197 = Array Subset(array=w4050, index (row)=0 ("index"), length (row)=4 ("length"), index (col)=0 ("index"), length (col)=1 ("length")) -> (w4045:T45)
          }
        }
        n2198 = feedback-in #16(w4011) -> ()
        n2199 = Split 1D Array(array=w4025, index=2) -> (first subarray=→"FFT 1":cluster{"f0":dbl, "df":dbl, "magnitude":dbl[]}[], second subarray=→"FFT 2":cluster{"f0":dbl, "df":dbl, "magnitude":dbl[]}[])
      }
    }
    n2200 = case "For plotting results of scanning MCL" shown="True" w3078 {
      tunnel: w3077 -> [_ w3463]
      tunnel: w2995 -> [_ w3559]
      tunnel: w3086 -> [_ _]
      tunnel: w2964 -> [_ w3533]
      tunnel: w2939 -> [_ w3464]
      tunnel: w2938 -> [_ w3437]
      frame False {
      }
      frame True {
        w3444 = u32 0 items=["Horizontal", "Vertical", "Central", "1st Diagonal", "2nd Diagonal"] ("Type of Symmetry")
        w3472 = u32 0 items=["Horizontal", "Vertical", "Central", "1st Diagonal", "2nd Diagonal"] ("Type of Symmetry")
        w3475 = u32 0 items=["Horizontal", "Vertical", "Central", "1st Diagonal", "2nd Diagonal"] ("Type of Symmetry")
        w3504 = u32 0 items=["Horizontal", "Vertical", "Central", "1st Diagonal", "2nd Diagonal"] ("Type of Symmetry")
        n2201 = Index Array(array=w3533, index=10) -> (element=w3539:waveform(dbl))
        n2202 = Index Array(array=w3533, index=11) -> (element=w3536:waveform(dbl))
        n2203 = local read "Cycles/step (MCL)"() -> (w3489:u64)
        n2204 = Index Array(array=w3533, index="Channel") -> (element=w3535:waveform(dbl))
        n2205 = Unbundle(w3437) -> ("New Image"=w3436:T2, "New Image"=w3435:T2, "New Image"=w3434:T2, "New Image"=w3433:T2)
        n2206 = Unbundle By Name(w3539) -> ("Y"=w3491:dbl[])
        n2207 = Unbundle By Name(w3536) -> ("Y"=w3493:dbl[])
        n2208 = Unbundle By Name(w3535) -> ("Y"=w3498:dbl[])
        n2209 = call "downsample 1D array - double.vi"("Ave N"=w3489, "Array In"=w3491) -> ("Array Out"=w3490:dbl[])  [unwired: 1 out]
        n2210 = call "downsample 1D array - double.vi"("Ave N"=w3489, "Array In"=w3493) -> ("Array Out"=w3492:dbl[])  [unwired: 1 out]
        n2211 = call "downsample 1D array - double.vi"("Ave N"=w3489, "Array In"=w3498) -> ("Array Out"=w3497:dbl[])  [unwired: 1 out]
        n2212 = feedback #17(w3559) -> (w3560:dbl[])
        n2213 = Build Array (concatenate)(w3560, w3559) -> (w3541:dbl[])
        n2214 = feedback #18(w3464) -> (w3466:dbl[])
        n2215 = Build Array (concatenate)(w3466, w3464) -> (w3465:dbl[])
        n2216 = local read "Scan steps (MCL)"() -> (w3446:u64)
        n2217 = Select(t=w3559, s=w3463, f=w3541) -> (s? t:f=w3545:dbl[])
        n2218 = feedback-in #17(w3545) -> ()
        n2219 = Select(t=w3464, s=w3463, f=w3465) -> (s? t:f=w3447:dbl[])
        n2220 = feedback-in #18(w3447) -> ()
        n2221 = local read "Scan lines (y)"() -> (w3432:u64)
        n2222 = local read "N APD Samp/step"() -> (w3448:dbl)
        n2223 = feedback #19(w3490) -> (w3547:dbl[])
        n2224 = Build Array (concatenate)(w3547, w3490) -> (w3538:dbl[])
        n2225 = feedback #20(w3497) -> (w3557:dbl[])
        n2226 = Build Array (concatenate)(w3557, w3497) -> (w3556:dbl[])
        n2227 = feedback #21(w3492) -> (w3549:dbl[])
        n2228 = Build Array (concatenate)(w3549, w3492) -> (w3550:dbl[])
        n2229 = Select(t=w3490, s=w3463, f=w3538) -> (s? t:f=w3494:dbl[])
        n2230 = feedback-in #19(w3494) -> ()
        n2231 = Select(t=w3497, s=w3463, f=w3556) -> (s? t:f=w3496:dbl[])
        n2232 = feedback-in #20(w3496) -> ()
        n2233 = Select(t=w3492, s=w3463, f=w3550) -> (s? t:f=w3495:dbl[])
        n2234 = feedback-in #21(w3495) -> ()
        n2235 = Multiply(x=w3446, y=u64 2) -> (x*y=w3431:u64)
        n2236 = call "integrate 1D array interval - double.vi"("Ave N"=w3448, "Array In"=w3447) -> ("Array Out"=w3459:dbl[])  [unwired: 1 out]
        n2237 = call "integrate 1D array interval - double.vi"("Ave N"=w3448, "Array In"=w3545) -> ("Array Out"=w3544:dbl[])  [unwired: 1 out]
        n2238 = Array Size(array=w3459) -> (size(s)=w3460:i32)
        n2239 = Array Size(array=w3544) -> (size(s)=w3546:i32)
        n2240 = Multiply(x=w3432, y=w3431) -> (x*y=w3462:u64)
        n2241 = Multiply(x=w3432, y=w3431) -> (x*y=w3554:u64)
        n2242 = call <vilib>:"Mean.vi"("X"=w3494) -> ("mean"=w3478:dbl)  [unwired: 1 out]
        n2243 = Subtract(x=w3462, y=w3460) -> (x-y=w3453:u64)
        n2244 = call <vilib>:"Mean.vi"("X"=w3496) -> ("mean"=w3483:dbl)  [unwired: 1 out]
        n2245 = call <vilib>:"Mean.vi"("X"=w3495) -> ("mean"=w3481:dbl)  [unwired: 1 out]
